vi "EXAMENLABOADELANTOMYRIO.vi"() -> ()   [LabVIEW 2018]
uses:
  CONTROLADELANTO.ctl
  <vilib>/myRIO/Express VI/Onboard IO/DI/DI Express VI.xnode
  <vilib>/myRIO/Instrument Drivers/Onboard IO/DIO/vis/Read.vi
  <vilib>/myRIO/Instrument Drivers/Onboard IO/DIO/DIO.lvlib
  <vilib>/myRIO/Common/Instrument Driver Framework/myRIO v1.0/DIO/typedefs/DIO Channels Enum.ctl
  <vilib>/myRIO/Common/Instrument Driver Framework/myRIO v1.0/DIO/typedefs/DIO Channels List.ctl
  <vilib>/myRIO/Common/Instrument Driver Framework/Utilities/typedefs/Generic FPGA Reference.ctl
  <vilib>/myRIO/Common/Instrument Driver Framework/Utilities/typedefs/myRIO v1.0 Reference.ctl
  <vilib>/myRIO/Common/Instrument Driver Framework/Utilities/typedefs/Hardware Version Enum.ctl
  <vilib>/myRIO/Common/Instrument Driver Framework/Utilities/typedefs/myRIO Generic Hardware Reference.ctl
  <vilib>/myRIO/Instrument Drivers/Onboard IO/DIO/typedefs/DIO Reference.ctl
  <vilib>/myRIO/Instrument Drivers/Onboard IO/DIO/vis/myRIO DIO Open.xnode
  <vilib>/myRIO/Common/Instrument Driver Framework/Utilities/vis/Is FPGA Ref Available.vi
  <vilib>/myRIO/Common/Instrument Driver Framework/myRIO v1.0/DIO/vis/myRIO v1.1 Open DIO.vi
  <vilib>/userdefined/High Color/nirio_resource_hc.ctl
panel:
  out "PTE H":i32
  out "ESTADO":T1
  in  "stop":bool
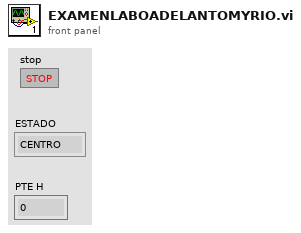
[diagram p1: front panel]
types:
  T1 = typedef "CONTROLADELANTO.ctl" = enum16{"CENTRO", "IZQUIERDA", "DERECHA", "VACENTROIZQUIERDA", "VACENTRODERECHA", "VAIZQUIERDA", "VADERECHA"}
  T2 = typedef "DIO.lvlib/DIO Reference.ctl" = cluster{"myRIO Reference":T3, "DIO Channels List":T7}
  T3 = typedef "myRIO Generic Hardware Reference.ctl" = cluster{"myRIO Model":T4, "myRIO Hardware Reference":T5}
  T4 = typedef "Hardware Version Enum.ctl" = enum16{"Unknown", "myRIO-1900", "myRIO-1950", "roboRIO", "NI ELVIS RIO CM", "ELVIS III"}
  T5 = typedef "myRIO v1.0 Reference.ctl" = cluster{"Generic FPGA Reference":T6, "Allow multiple opens":bool}
  T6 = typedef "Generic FPGA Reference.ctl" = refnum<k20>
  T7 = typedef "DIO Channels List.ctl" = T8[]
  T8 = typedef "DIO Channels Enum.ctl" = enum16{"Not Connected", "C/DIO0", "C/DIO1", "C/DIO2", "C/DIO3", "C/DIO4", "C/DIO5", "C/DIO6", "C/DIO7", "A/DIO0", "A/DIO1", "A/DIO2", "A/DIO3", "A/DIO4", "A/DIO5", "A/DIO6", "A/DIO7", "A/DIO8", "A/DIO9", "A/DIO10", "A/DIO11", "A/DIO12", "A/DIO13", "A/DIO14", "A/DIO15", "A/DIO16", "A/DIO17", "A/DIO18", "A/DIO19", "B/DIO0", "B/DIO1", "B/DIO2", "B/DIO3", "B/DIO4", "B/DIO5", "B/DIO6", "B/DIO7", "B/DIO8", "B/DIO9", "B/DIO10", "B/DIO11", "B/DIO12", "B/DIO13", "B/DIO14", "B/DIO15", "B/DIO16", "B/DIO17", "B/DIO18", "B/DIO19", "LED0", "LED1", "LED2", "LED3", "Button0", "DIO/DIO0", "DIO/DIO1", "DIO/DIO2", "DIO/DIO3", "DIO/DIO4", "DIO/DIO5", "DIO/DIO6", "DIO/DIO7", "DIO/DIO8", "DIO/DIO9", "SPI/CS0", "SPI/CS1", "SPI/CS2", "SPI/CS3", "LED RADIO (Green)", "LED RADIO (Red)", "LED COMM (Green)", "LED COMM (Red)", "LED MODE (Green)", "LED MODE (Red)"}
  T9 = typedef "nirio_resource_hc.ctl" = tag
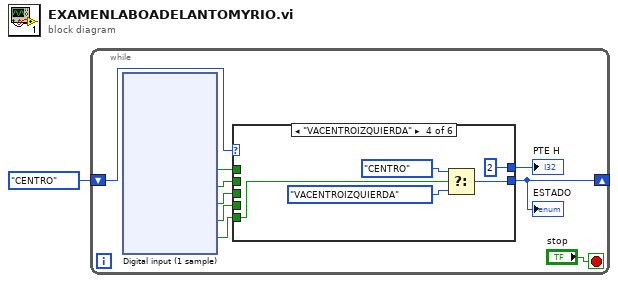
[diagram p0: block diagram]
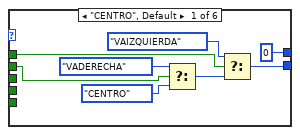
[diagram p2: hidden frame]
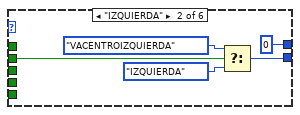
[diagram p3: hidden frame]
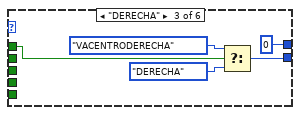
[diagram p4: hidden frame]
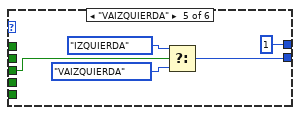
[diagram p5: hidden frame]
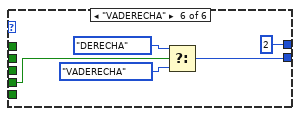
[diagram p6: hidden frame]
diagram:
  n1 = while {
    shift-right: [w2] -> _
    shift-left: CONTROLADELANTO."CENTRO" -> [w3]
    stop <- "stop" stop-if-true
    n2 = xnode "Digital input (1 sample)"() -> ("IZQUIERDA (A/DIO0 (Pin 11))"=w6:bool, "DERECHA (A/DIO1 (Pin 13))"=w4:bool, "SI (A/DIO2 (Pin 15))"=w8:bool, "SD (A/DIO3 (Pin 17))"=w7:bool, "SC (A/DIO4 (Pin 19))"=w5:bool)  [unwired: 1 in, 1 out]
    n3 = case shown="\"VACENTROIZQUIERDA\"" w3 {
      tunnel: w6 -> [w57 _ w67 _ _ _]
      tunnel: w4 -> [w55 w61 _ _ _ _]
      tunnel: [w51 w59 w65 w70 w74 w79] -> w2
      tunnel: [0 0 0 2 1 2] -> w9
      tunnel: w8 -> [_ _ _ _ w77 _]
      tunnel: w5 -> [_ _ _ w72 _ _]
      tunnel: w7 -> [_ _ _ _ _ w82]
      frame "CENTRO", Default {
        n4 = Select(t=CONTROLADELANTO."VADERECHA", s=w55, f=CONTROLADELANTO."CENTRO") -> (s? t:f=w56:T1)
        n5 = Select(t=CONTROLADELANTO."VAIZQUIERDA", s=w57, f=w56) -> (s? t:f=w51:T1)
      }
      frame "IZQUIERDA" {
        n6 = Select(t=CONTROLADELANTO."VACENTROIZQUIERDA", s=w61, f=CONTROLADELANTO."IZQUIERDA") -> (s? t:f=w59:T1)
      }
      frame "DERECHA" {
        n7 = Select(t=CONTROLADELANTO."VACENTRODERECHA", s=w67, f=CONTROLADELANTO."DERECHA") -> (s? t:f=w65:T1)
      }
      frame "VACENTROIZQUIERDA" {
        n8 = Select(t=CONTROLADELANTO."CENTRO", s=w72, f=CONTROLADELANTO."VACENTROIZQUIERDA") -> (s? t:f=w70:T1)
      }
      frame "VAIZQUIERDA" {
        n9 = Select(t=CONTROLADELANTO."IZQUIERDA", s=w77, f=CONTROLADELANTO."VAIZQUIERDA") -> (s? t:f=w74:T1)
      }
      frame "VADERECHA" {
        n10 = Select(t=CONTROLADELANTO."DERECHA", s=w82, f=CONTROLADELANTO."VADERECHA") -> (s? t:f=w79:T1)
      }
    }
    "ESTADO" <- w2
    "PTE H" <- w9
  }
